vi "Asylum_SetSTFC.vi"(5 "eventString":string, 6 "trigger":cluster{"Value":dbl, "greaterOrLesser":dbl}, 7 "z":cluster{"Start":dbl, "End":dbl}, 8 "error in (no error)":errorcluster, 9 "inChannelString":string, 10 "time":dbl, 11 "Application":refnum<k7>) -> (0 "error out":errorcluster, 3 "Application":refnum<k7>)   [LabVIEW 2019]
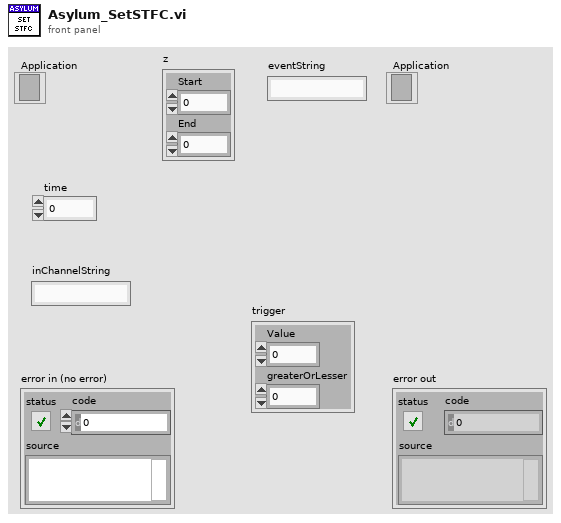
[diagram p1: front panel]
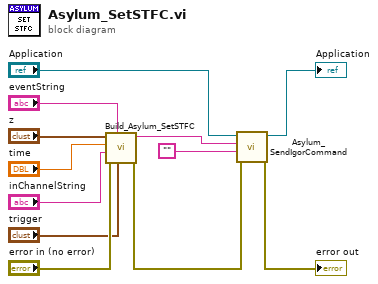
[diagram p0: block diagram]
diagram:
  n1 = call "Build_Asylum_SetSTFC.vi"("trigger"="trigger", "eventString"="eventString", "error in (no error)"="error in (no error)", "inChannelString"="inChannelString", "time"="time", "z"="z") -> ("error out"=w12:errorcluster, "Command"=w10:string)  [unwired: 4 in]
  n2 = call "Asylum_SendIgorCommand.vi"("error in (no error)"=w12, "Format"="", "command"=w10, "Application In"="Application") -> ("error out"=→"error out":errorcluster, "Application Out"=→"Application":refnum<k7>)  [unwired: 4 in, 2 out]
